vi "single.vi"(2 "error in (no error)":errorcluster, 3 "OSC in":refnum<visa-resource-name>) -> (0 "error out":errorcluster, 1 "OSC out":refnum<visa-resource-name>)   [LabVIEW 2016]
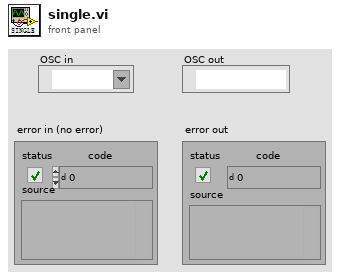
[diagram p1: front panel]
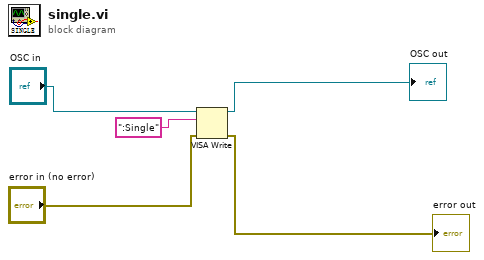
[diagram p0: block diagram]
diagram:
  n1 = VISA Write(VISA resource name="OSC in", write buffer=":Single", error in (no error)="error in (no error)") -> (VISA resource name out=→"OSC out":refnum<visa-resource-name>, error out=→"error out":errorcluster)  [unwired: 1 out]
